vi "AlgorithmRightGoal.vi"(6 "MatchBallY":dbl, 7 "MatchBallX":dbl, 8 "D2 Y COM":dbl, 9 "D2 X COM":dbl, 10 "D1Y COM":dbl, 11 "D1 X COM":dbl) -> (0 "min x3":dbl, 1 "aS":dbl, 2 "min x2":dbl, 3 "aRW":dbl, 4 "min x":dbl, 5 "Theta LG,LW":dbl)   [LabVIEW 2014]
panel:
  out "xD2BotS":dbl
  out "xD2ComS":dbl
  out "xD1BotS":dbl
  out "xD1ComS":dbl
  out "xD2BotR":dbl
  out "xD2ComR":dbl
  out "xD1BotR":dbl
  out "xD1ComR":dbl
  out "D2 X Bot fit 2":dbl
  out "D2 X Com fit":dbl
  out "D1 X Bot fit":dbl
  out "D1 X Com fit":dbl
  # "LOGIC"
  # "Left Goal"
  # "STRAIGHT"
  # "Left wall"
  # "Right Wall"
  # "Straight"
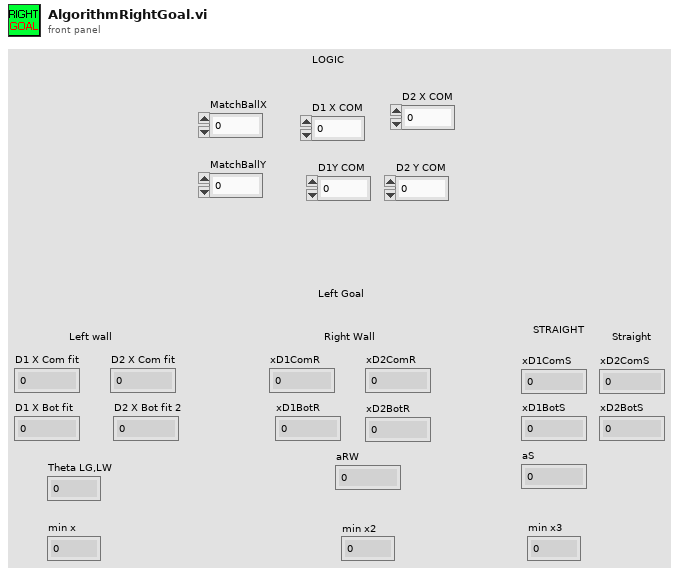
[diagram p1: front panel]
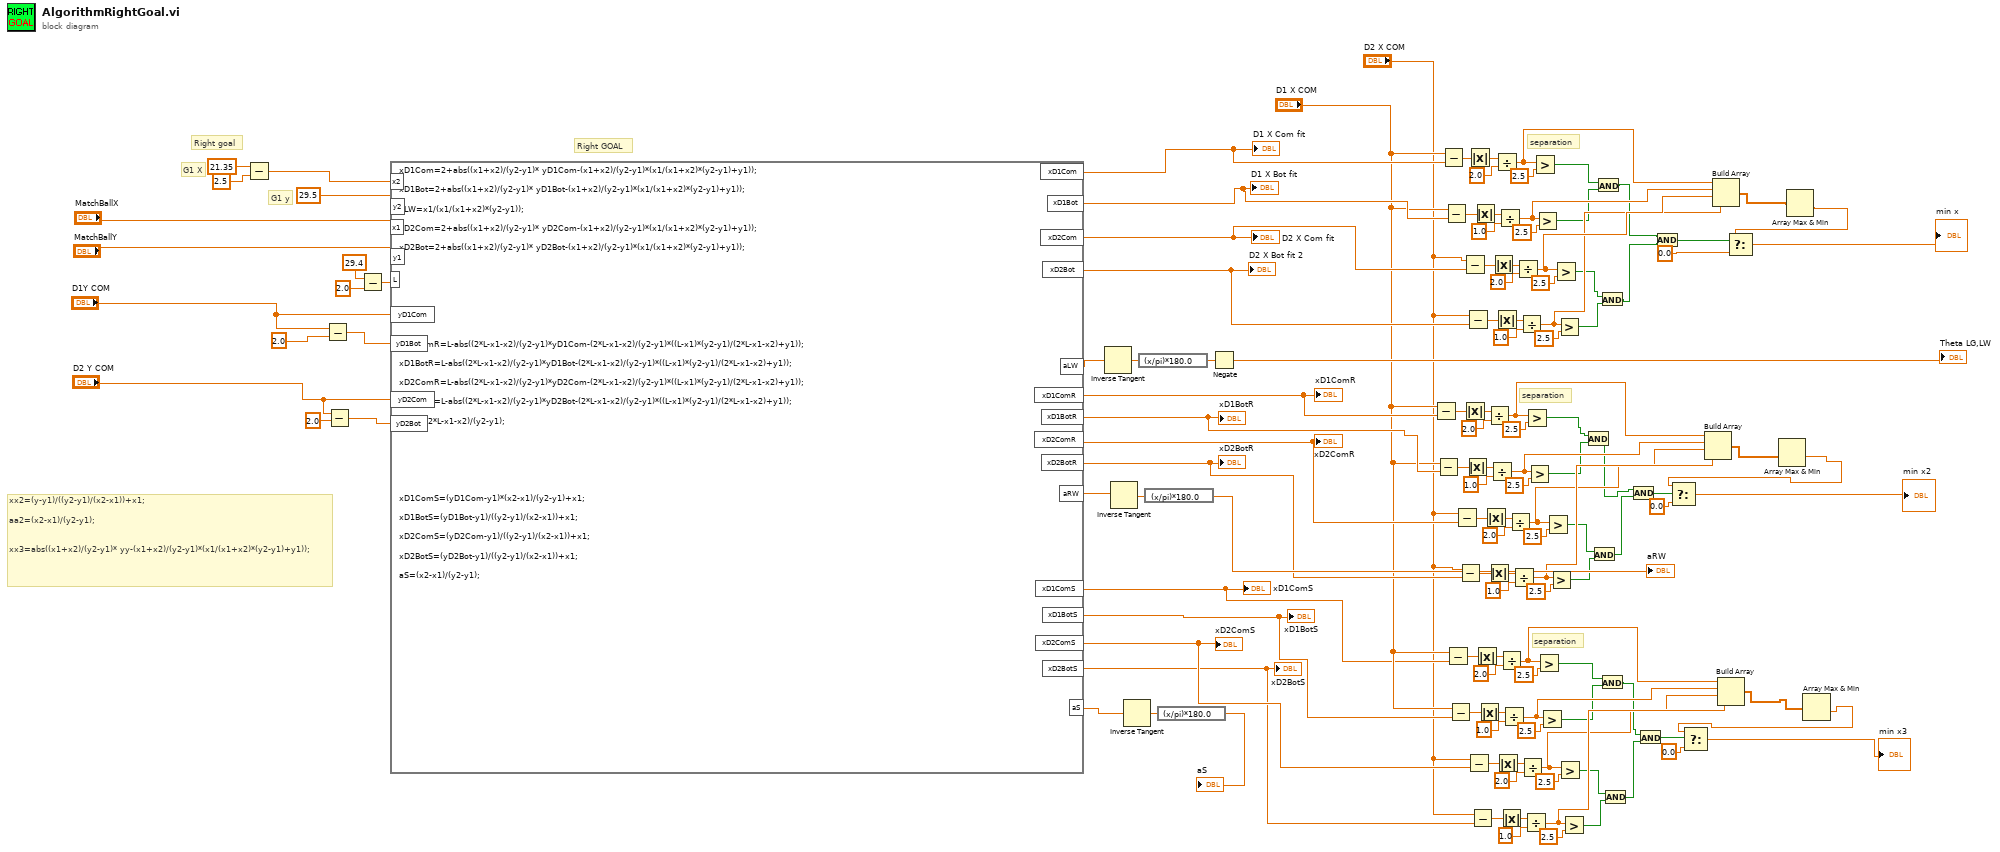
[diagram p0: block diagram]
diagram:
  # "separation"
  # "separation"
  # "separation"
  # "Right GOAL"
  # "xx2=(y-y1)/((y2-y1)/(x2-x1))+x1;\n\naa2=(x2-x1)/(y2-y1);\n\n\nxx3=abs((x1+x2)/(y2-y1)* yy-(x1+x2)/(y2-y1)*(x1/(x1+x2)*(y2-y1)+y1));"
  # "Right goal"
  # "G1 y"
  # "G1 X"
  n1 = Subtract(x=21.35, y=2.5) -> (x-y=w127:dbl)
  n2 = Subtract(x="D1Y COM", y=2.0) -> (x-y=w122:dbl)
  n3 = Subtract(x="D2 Y COM", y=2.0) -> (x-y=w117:dbl)
  n4 = Subtract(x=29.4 ("input variable"), y=2.0) -> (x-y=w2:dbl)
  n5 = formula code="xD1Com=2+abs((x1+x2)/(y2-y1)* yD1Com-(x1+x2)/(y2-y1)*(x1/(x1+x2)*(y2-y1)+y1));\n\nxD1Bot=2+abs((x1+x2)/(y2-y1)* yD1Bot-(x1+x2)/(y2-y1)*(x1/(x1+x2)*(y2-y1)+y1));\n\naLW=x1/(x1/(x1+x2)*(y2-y1));\n\nxD2Com=2+abs((x1+x2)/(y2-y1)* yD2Com-(x1+x2)/(y2-y1)*(x1/(x1+x2)*(y2-y1)+y1));\n\nxD2Bot=2+abs((x1+x2)/(y2-y1)* yD2Bot-(x1+x2)/(y2-y1)*(x1/(x1+x2)*(y2-y1)+y1));\n\n\n\n\n\n\n\n\n\nxD1ComR=L-abs((2*L-x1-x2)/(y2-y1)*yD1Com-(2*L-x1-x2)/(y2-y1)*((L-x1)*(y2-y1)/(2*L-x1-x2)+y1));\n\nxD1BotR=L-abs((2*L-x1-x2)/(y2-y1)*yD1Bot-(2*L-x1-x2)/(y2-y1)*((L-x1)*(y2-y1)/(2*L-x1-x2)+y1));\n\nxD2ComR=L-abs((2*L-x1-x2)/(y2-y1)*yD2Com-(2*L-x1-x2)/(y2-y1)*((L-x1)*(y2-y1)/(2*L-x1-x2)+y1));\n\nxD2BotR=L-abs((2*L-x1-x2)/(y2-y1)*yD2Bot-(2*L-x1-x2)/(y2-y1)*((L-x1)*(y2-y1)/(2*L-x1-x2)+y1));\n\naRW=(2*L-x1-x2)/(y2-y1);\n\n\n\n\n\n\n\nxD1ComS=(yD1Com-y1)*(x2-x1)/(y2-y1)+x1;\n\nxD1BotS=(yD1Bot-y1)/((y2-y1)/(x2-x1))+x1;\n\nxD2ComS=(yD2Com-y1)/((y2-y1)/(x2-x1))+x1;\n\nxD2BotS=(yD2Bot-y1)/((y2-y1)/(x2-x1))+x1;\n\naS=(x2-x1)/(y2-y1);"("x1"="MatchBallX", "x2"=w127, "y2"=29.5, "y1"="MatchBallY", "yD1Com"="D1Y COM", "yD2Com"="D2 Y COM", "yD1Bot"=w122, "yD2Bot"=w117, "L"=w2) -> ("xD1Com"=w110:dbl, "aLW"=w125:dbl, "xD1Bot"=w96:dbl, "xD2Com"=w101:dbl, "xD2Bot"=w91:dbl, "xD1ComR"=w64:dbl, "xD1BotR"=w63:dbl, "xD2ComR"=w62:dbl, "xD2BotR"=w61:dbl, "aRW"=w115:dbl, "xD1ComS"=w38:dbl, "aS"=w111:dbl, "xD1BotS"=w37:dbl, "xD2BotS"=w35:dbl, "xD2ComS"=w36:dbl)
  "D1 X Com fit" <- w110
  "D1 X Bot fit" <- w96
  "D2 X Com fit" <- w101
  "D2 X Bot fit 2" <- w91
  "xD1ComR" <- w64
  "xD1BotR" <- w63
  "xD2ComR" <- w62
  "xD2BotR" <- w61
  "xD1ComS" <- w38
  "xD1BotS" <- w37
  "xD2ComS" <- w36
  "xD2BotS" <- w35
  n6 = Inverse Tangent(1:w125) -> (0:w126:dbl)
  n7 = Inverse Tangent(1:w115) -> (0:w116:dbl)
  n8 = Inverse Tangent(1:w111) -> (0:w112:dbl)
  n9 = expression code="(x/pi)*180.0" ("radians to degrees")(w126) -> (w123:dbl)
  n10 = expression code="(x/pi)*180.0" ("radians to degrees")(w116) -> (→"aRW":dbl)
  n11 = expression code="(x/pi)*180.0" ("radians to degrees")(w112) -> (→"aS":dbl)
  n12 = Negate(x=w123) -> (-x=→"Theta LG,LW":dbl)
  n13 = Subtract(x="D1 X COM", y=w64) -> (x-y=w65:dbl)
  n14 = Subtract(x="D1 X COM", y=w63) -> (x-y=w76:dbl)
  n15 = Subtract(x="D1 X COM", y=w110) -> (x-y=w109:dbl)
  n16 = Subtract(x="D1 X COM", y=w96) -> (x-y=w97:dbl)
  n17 = Subtract(x="D1 X COM", y=w38) -> (x-y=w40:dbl)
  n18 = Subtract(x="D1 X COM", y=w37) -> (x-y=w51:dbl)
  n19 = Subtract(x="D2 X COM", y=w62) -> (x-y=w72:dbl)
  n20 = Subtract(x="D2 X COM", y=w61) -> (x-y=w77:dbl)
  n21 = Subtract(x="D2 X COM", y=w101) -> (x-y=w102:dbl)
  n22 = Absolute Value(x=w65) -> (abs(x)=w66:dbl)
  n23 = Absolute Value(x=w76) -> (abs(x)=w75:dbl)
  n24 = Subtract(x="D2 X COM", y=w91) -> (x-y=w95:dbl)
  n25 = Subtract(x="D2 X COM", y=w36) -> (x-y=w47:dbl)
  n26 = Absolute Value(x=w109) -> (abs(x)=w108:dbl)
  n27 = Subtract(x="D2 X COM", y=w35) -> (x-y=w52:dbl)
  n28 = Absolute Value(x=w97) -> (abs(x)=w98:dbl)
  n29 = Absolute Value(x=w40) -> (abs(x)=w41:dbl)
  n30 = Absolute Value(x=w51) -> (abs(x)=w50:dbl)
  n31 = Absolute Value(x=w72) -> (abs(x)=w71:dbl)
  n32 = Divide(x=w66, y=2.0) -> (x/y=w82:dbl)
  n33 = Absolute Value(x=w77) -> (abs(x)=w78:dbl)
  n34 = Divide(x=w75, y=1.0) -> (x/y=w83:dbl)
  n35 = Absolute Value(x=w102) -> (abs(x)=w103:dbl)
  n36 = Divide(x=w108, y=2.0) -> (x/y=w89:dbl)
  n37 = Absolute Value(x=w95) -> (abs(x)=w94:dbl)
  n38 = Absolute Value(x=w47) -> (abs(x)=w46:dbl)
  n39 = Divide(x=w98, y=1.0) -> (x/y=w88:dbl)
  n40 = Divide(x=w41, y=2.0) -> (x/y=w57:dbl)
  n41 = Absolute Value(x=w52) -> (abs(x)=w53:dbl)
  n42 = Divide(x=w50, y=1.0) -> (x/y=w58:dbl)
  n43 = Divide(x=w71, y=2.0) -> (x/y=w84:dbl)
  n44 = Divide(x=w78, y=1.0) -> (x/y=w85:dbl)
  n45 = Divide(x=w103, y=2.0) -> (x/y=w87:dbl)
  n46 = Divide(x=w94, y=1.0) -> (x/y=w86:dbl)
  n47 = Divide(x=w46, y=2.0) -> (x/y=w59:dbl)
  n48 = Divide(x=w53, y=1.0) -> (x/y=w60:dbl)
  n49 = Greater?(x=w82, y=2.5) -> (0:w21:bool)
  n50 = Greater?(x=w83, y=2.5) -> (0:w20:bool)
  n51 = Greater?(x=w89, y=2.5) -> (0:w26:bool)
  n52 = Greater?(x=w88, y=2.5) -> (0:w25:bool)
  n53 = Greater?(x=w57, y=2.5) -> (0:w16:bool)
  n54 = Greater?(x=w58, y=2.5) -> (0:w15:bool)
  n55 = Greater?(x=w84, y=2.5) -> (0:w19:bool)
  n56 = Greater?(x=w85, y=2.5) -> (0:w18:bool)
  n57 = Greater?(x=w87, y=2.5) -> (0:w30:bool)
  n58 = Greater?(x=w86, y=2.5) -> (0:w29:bool)
  n59 = Greater?(x=w59, y=2.5) -> (0:w13:bool)
  n60 = Greater?(x=w60, y=2.5) -> (0:w12:bool)
  n61 = And(x=w21, y=w20) -> (x .and. y?=w22:bool)
  n62 = And(x=w19, y=w18) -> (x .and. y?=w17:bool)
  n63 = And(x=w26, y=w25) -> (x .and. y?=w24:bool)
  n64 = And(x=w30, y=w29) -> (x .and. y?=w27:bool)
  n65 = And(x=w16, y=w15) -> (x .and. y?=w14:bool)
  n66 = And(x=w13, y=w12) -> (x .and. y?=w11:bool)
  n67 = And(x=w22, y=w17) -> (x .and. y?=w23:bool)
  n68 = And(x=w14, y=w11) -> (x .and. y?=w10:bool)
  n69 = And(x=w24, y=w27) -> (x .and. y?=w28:bool)
  n70 = Build Array(w82, w83, w84, w85) -> (w7:dbl[])
  n71 = Build Array(w89, w88, w87, w86) -> (w9:dbl[])
  n72 = Build Array(w57, w58, w59, w60) -> (w5:dbl[])
  n73 = Array Max & Min(array=w7) -> (min value=w6:dbl)  [unwired: 3 out]
  n74 = Select(t=w6, s=w23, f=0.0 ("y")) -> (s? t:f=→"min x2":dbl)
  n75 = Array Max & Min(array=w9) -> (min value=w8:dbl)  [unwired: 3 out]
  n76 = Select(t=w8, s=w28, f=0.0 ("y")) -> (s? t:f=→"min x":dbl)
  n77 = Array Max & Min(array=w5) -> (min value=w4:dbl)  [unwired: 3 out]
  n78 = Select(t=w4, s=w10, f=0.0 ("y")) -> (s? t:f=→"min x3":dbl)
